vi "Andor_LiveGraph.vi"() -> ()   [LabVIEW 2019]
panel:
  in  "Booléen":bool
  in  "Show Avg":bool
  in  "Avg Val":i32=1 min=1 max=10000 step=1
  out "Data":T1
  in  "error in (no error)":errorcluster caption="entrée d'erreur (pas d'erreur)"
  out "Graph":T2(graph)
  out "Ch2":dbl
  out "Ch1":dbl
  out "error out":errorcluster caption="sortie d'erreur"
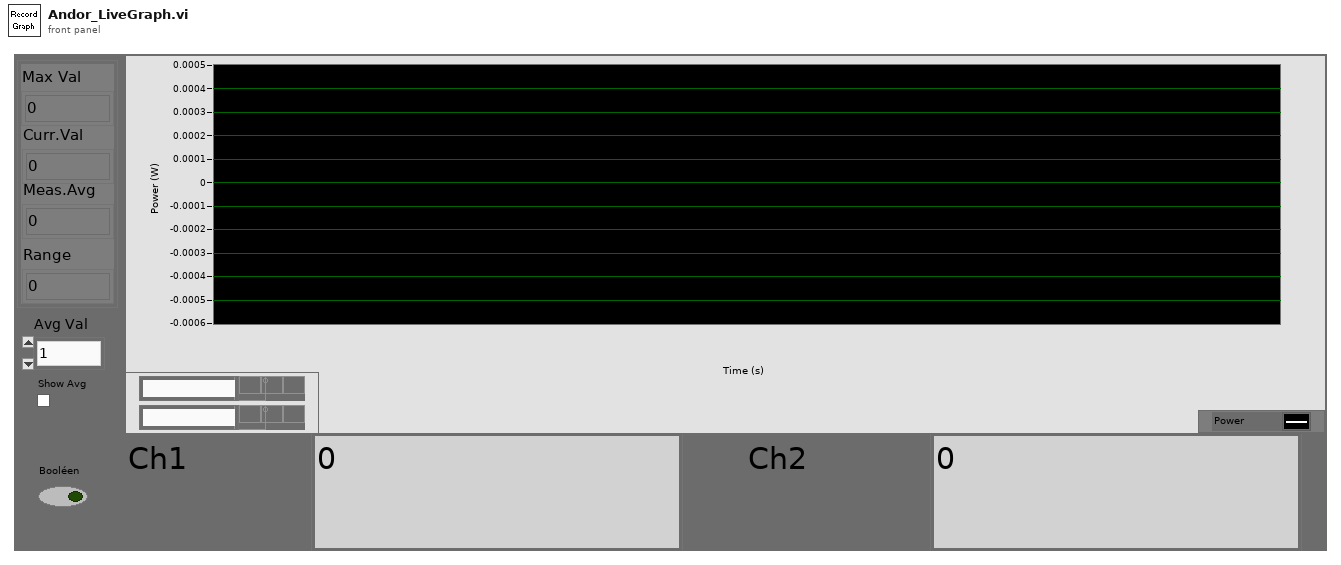
[diagram p1: front panel]
types:
  T1 = cluster{"Max Val":dbl, "Curr.Val":dbl, "Meas.Avg":dbl, "Range":dbl}
  T2 = cluster{dbl, "Resolution (ns)":dbl, "Histogram":dbl[]}
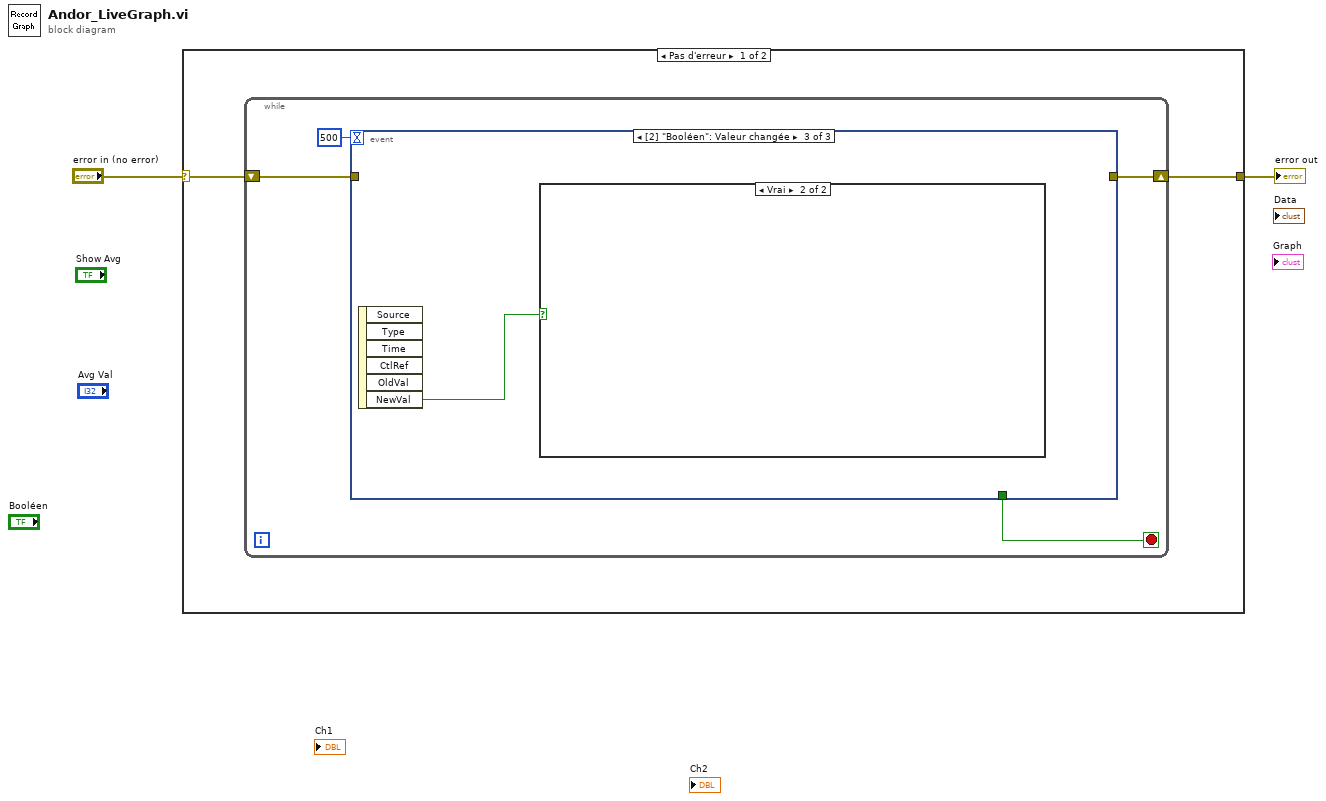
[diagram p0: block diagram]
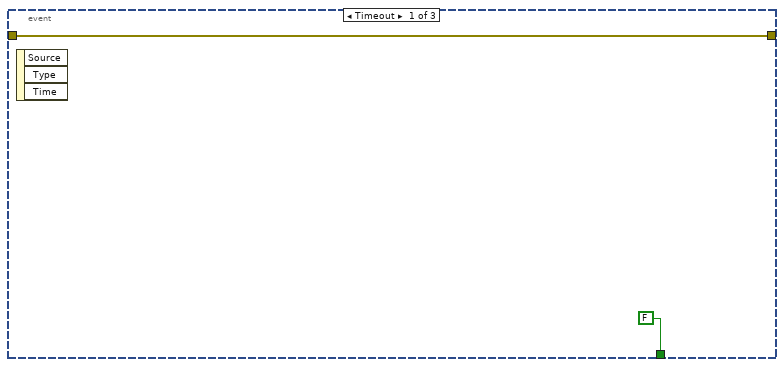
[diagram p2: hidden frame]
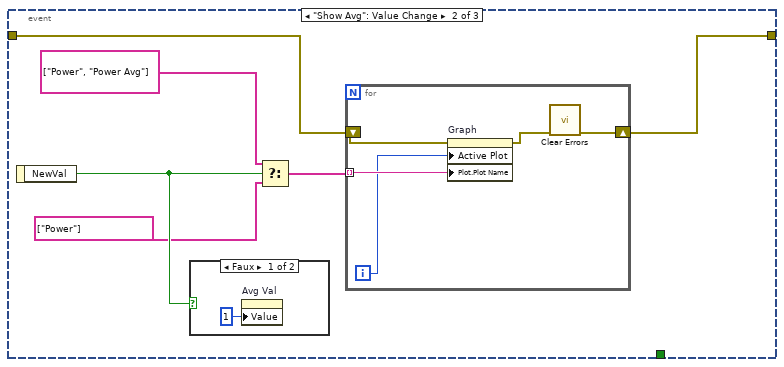
[diagram p3: hidden frame]
diagram:
  n1 = case shown="Pas d'erreur" "error in (no error)" {
    selector: "error in (no error)" -> [w3 w24]
    tunnel: [w4 w24] -> w2
    frame No Error {
      n2 = while {
        shift-right: [w7] -> w4
        shift-left: w3 -> [w6]
        stop <- w5 stop-if-true
        n3 = event shown="[2] \"Booléen\": Valeur changée" {
          selector: _ -> [_ _ _]
          dyn-events: _ -> [_ _ _]
          timeout: 500 -> [_ _ _]
          tunnel: [w10 w13 _] -> w7
          tunnel: w6 -> [w10 w14 _]
          tunnel: [FALSE _ _] -> w5
          event Timeout {
            n4 = event-data() -> ()  [unwired: 1 in, 3 out]
          }
          event "Show Avg": Value Change {
            n5 = event-data() -> ("NewVal"=w12:bool)  [unwired: 1 in]
            n6 = case shown="Faux" w12 {
              frame False {
                n7 = property on="Avg Val" class="NumNb (strict)"("Value"=1 ("Avg Val")) -> ()  [unwired: 2 in, 2 out]
              }
              frame True {
              }
            }
            n8 = Select(t=string[] ["Power", "Power Avg"], s=w12, f=string[] ["Power"]) -> (s? t:f=w15:string[])
            n9 = for {
              tunnel: w15 -> [w22] mode=indexing
              shift-right: [w19] -> w13
              shift-left: w14 -> [w21]
              i -> [w18]
              n10 = property on="Graph" class="GraphWF (strict)"(error in=w21, "Active Plot"=w18, "Plot.Plot Name"=w22) -> (error out=w20:errorcluster)  [unwired: 1 in, 1 out]
              n11 = call <vilib>:"Clear Errors.vi"("error in (no error)"=w20) -> ("error out"=w19:errorcluster)  [unwired: 5 in, 1 out]
            }
          }
          event "Booléen": Value Change {
            n12 = event-data() -> ("NewVal"=w23:bool)  [unwired: 1 in, 5 out]
            n13 = case shown="Vrai" w23 {
              frame False {
              }
              frame True {
              }
            }
          }
        }
      }
    }
    frame Error {
    }
  }
  "error out" <- w2
